vi "Configure Filter Constant.vi"(5 "Retry Attempts (0)":i32 min=0, 7 "Unit Address (-1)":i32=-1, 8 "error in (no error)":errorcluster, 10 "Filter Constant":T2, 11 "VISA resource name (in)":refnum<visa-resource-name>) -> (0 "error out":errorcluster, 2 "Response Cluster":T1 {"Command ID" format="%x"}, 3 "VISA resource name (out)":refnum<visa-resource-name>)   [LabVIEW 2020, in "Omega Platinum Series.lvlib"]
doc: "Changes the filter constant to the given value from the Filter Constant enum typedef."
uses:
  <instrlib>/RxnRover/OmegaPlatinumSeriesDriver/Omega Platinum Series.lvlib
  <instrlib>/RxnRover/OmegaPlatinumSeriesDriver/Public/Type Defs/Filter Constant.ctl
  <instrlib>/RxnRover/OmegaPlatinumSeriesDriver/Public/Type Defs/Response.ctl
panel:
  out "Command":string
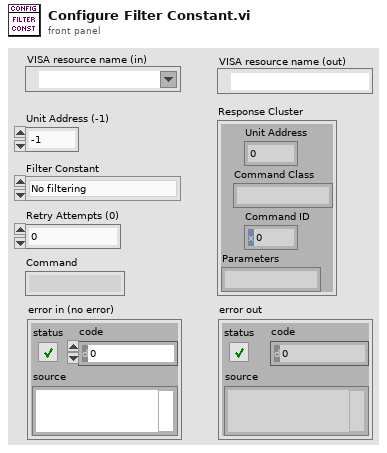
[diagram p1: front panel]
types:
  T1 = typedef "Omega Platinum Series.lvlib/Response.ctl" = cluster{"Unit Address":i32, "Command Class":string, "Command ID":u32, "Parameters":string}
  T2 = typedef "Omega Platinum Series.lvlib/Filter Constant.ctl" = enum16{"No filtering", "X 2 filtering", "X 4 filtering", "X 8 filtering", "X 16 filtering", "X 32 filtering", "X 64 filtering", "X 128 filtering"}
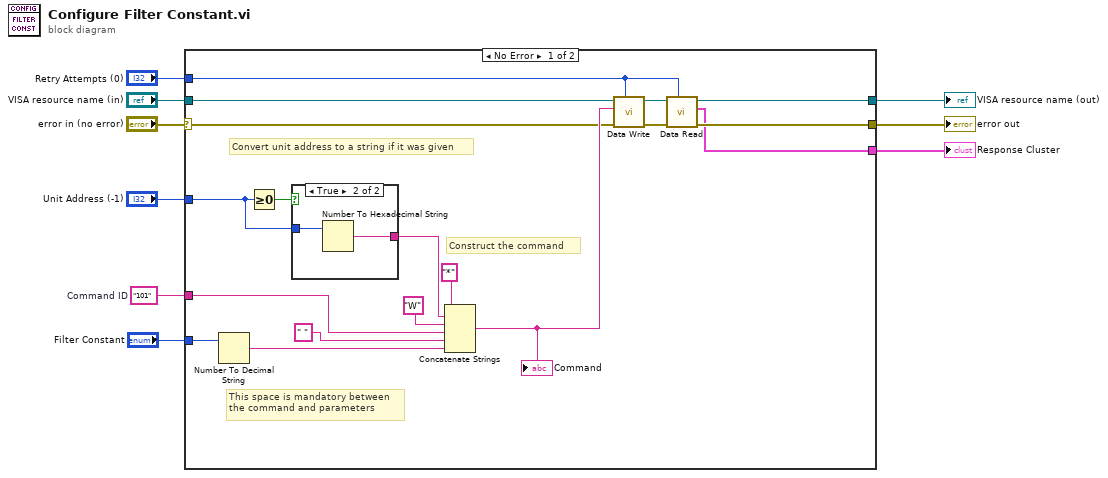
[diagram p0: block diagram]
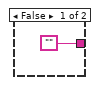
[diagram p2: hidden frame]
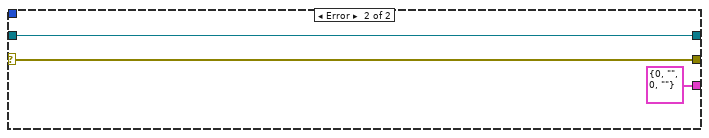
[diagram p3: hidden frame]
diagram:
  w8 = "101"  # Command ID
  n1 = case shown="No Error" "error in (no error)" {
    selector: "error in (no error)" -> [w20 w33]
    tunnel: "Filter Constant" -> [w27 _]
    tunnel: w8 -> [w13 _]
    tunnel: "Unit Address (-1)" -> [w24 _]
    tunnel: [w16 w33] -> w5
    tunnel: "VISA resource name (in)" -> [w22 w32]
    tunnel: [w17 w32] -> w3
    tunnel: [w15 T1 {"Unit Address"=0, "Command Class"="", "Command ID"=0, "Parameters"=""} ("Response Cluster")] -> w2
    tunnel: "Retry Attempts (0)" -> [w10 _]
    frame No Error {
      # "This space is mandatory between\nthe command and parameters"
      # "Convert unit address to a string if it was given"
      # "Construct the command"
      n2 = Number To Decimal String(number=w27) -> (decimal integer string=w12:string)  [unwired: 1 in]
      n3 = Greater Or Equal To 0?(x=w24) -> (x >= 0?=w26:bool)
      n4 = case shown="True" w26 {
        tunnel: w24 -> [_ w30]
        tunnel: ["" w29] -> w23
        frame False {
        }
        frame True {
          n5 = Number To Hexadecimal String(2:w30) -> (0:w29:string)  [unwired: 1 in]
        }
      }
      n6 = Concatenate Strings("*" ("string"), w23, "W" ("string"), w13, " " ("string"), w12) -> (w21:string)
      "Command" <- w21
      n7 = call <instrlib>:"Data Write.vi"("Retry Attempts (0)"=w10, "error in (no error)"=w20, "Command"=w21, "VISA Refnum in"=w22) -> ("error out"=w19:errorcluster, "VISA Refnum out"=w18:refnum<visa-resource-name>)  [unwired: 6 in]
      n8 = call <instrlib>:"Data Read.vi"("Retry Attempts (0)"=w10, "error in (no error)"=w19, "VISA Refnum in"=w18) -> ("error out"=w16:errorcluster, "Response Cluster"=w15:T1, "VISA Refnum out"=w17:refnum<visa-resource-name>)  [unwired: 5 in, 1 out]
    }
    frame Error {
    }
  }
  "error out" <- w5
  "VISA resource name (out)" <- w3
  "Response Cluster" <- w2
